vi "Scale Volt to Temp.vi"(1 "Input Value (V)":dbl format="%0.2f") -> (0 "Output Value (degC)":dbl format="%0.2f")   [LabVIEW 2017]
uses:
  <vilib>/Analysis/NI_AALPro.lvlib
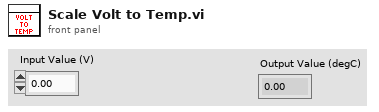
[diagram p1: front panel]
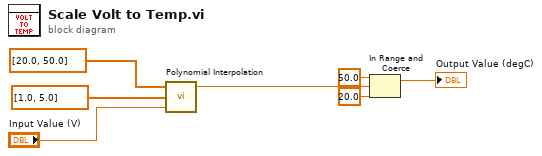
[diagram p0: block diagram]
diagram:
  n1 = call <vilib>:"Polynomial Interpolation.vi"("x value"="Input Value (V)", "X"=dbl[] [1.0, 5.0] ("Y"), "Y"=dbl[] [20.0, 50.0] ("X")) -> ("interpolation value"=w2:dbl)  [unwired: 2 out]
  n2 = In Range and Coerce(upper limit=50.0, x=w2, lower limit=20.0) -> (coerced(x)=→"Output Value (degC)":dbl)  [unwired: 1 out]
